vi "补偿电阻RsRp计算.vi"(6 "I":dbl=1.5244, 8 "A":dbl, 9 "压力点个数":dbl=3.0, 10 "检定次数":dbl=1.0, 11 "实时测量数据":string[][](array[string])=[["时间", "温度（℃）", "压力（KPa）", "电压1（V）", "桥压1（V）", "电压2（V）", "桥压2（V）", "电压3（V）", "桥压3（V）", "电压4（V）", "桥压4（V）", "电压5（V）", "桥压5（V）"], ["", "", "1", " ", "2", " ", "3", " ", "4", " ", "", "", ""], ["", "", "正行程", "", "", "", "", "", "", "", "", "", ""], ["17:06:40", "11.900000", "199.921", "-6.32\n-6.32\n", "7.8325\n", "-3.0-6.299\n67000E-6", "-2.844000E-6", "-3.300000E-6", "-3.109000E-6", "-3.045000E-6", "-2.897000E-6", "", ""], ["17:07:13", "12.000000", "299.9351", "51.474", "7.8338", "-3.013000E-6", "-3.491000E-6", "-2.918000E-6", "-3.332000E-6", "-2.780000E-6", "-3.204000E-6", "", ""], ["17:07:36", "12.000000", "399.96", "110.353", "7.8346", "-3.120000E-6", "-3.289000E-6", "-2.960000E-6", "-3.141000E-6", "-3.385000E-6", "-2.844000E-6", "", ""], ["", "", "反行程", "", "", "", "", "", "", "", "", "", ""], ["17:08:20", "12.000000", "400.0285", "110.353", "7.8346", "-3.120000E-6", "-3.342000E-6", "-3.162000E-6", "-3.194000E-6", "-3.056000E-6", "-3.194000E-6", "", ""], ["17:08:45", "12.000000", "300.0653", "52.283", "7.8332", "-3.342000E-6", "-3.321000E-6", "-3.013000E-6", "-3.311000E-6", "-3.300000E-6", "-3.162000E-6", "", ""], ["17:09:22", "12.000000", "200.0595", "-6.299", "7.8346", "-2.907000E-6", "-3.194000E-6", "-3.257000E-6", "-3.204000E-6", "-3.077000E-6", "-2.971000E-6", "", ""], ["", "", "正行程", "", "", "", "", "", "", "", "", "", ""], ["17:13:30", "12.100000", "199.9466", "-7.532", "8.8568", "-3.671000E-6", "-3.353000E-6", "-3.799000E-6", "-3.565000E-6", "-3.746000E-6", "-3.374000E-6", "", ""], ["17:13:53", "12.100000", "299.95", "53.539", "8.8574", "-3.311000E-6", "-3.502000E-6", "-3.364000E-6", "-3.618000E-6", "-3.120000E-6", "-3.406000E-6", "", ""], ["17:14:26", "12.100000", "399.8962", "116.27", "8.8567", "-3.756000E-6", "-3.830000E-6", "-3.427000E-6", "-3.597000E-6", "-3.777000E-6", "-3.576000E-6", "", ""], ["", "", "反行程", "", "", "", "", "", "", "", "", "", ""], ["17:15:01", "12.100000", "399.9835", "116.27", "8.8567", "-3.395000E-6", "-3.289000E-6", "-3.120000E-6", "-3.502000E-6", "-3.427000E-6", "-3.353000E-6", "", ""], ["17:15:38", "12.100000", "299.9459", "54.318", "8.8552", "-3.512000E-6", "-3.650000E-6", "-3.809000E-6", "-3.480000E-6", "-3.300000E-6", "-3.767000E-6", "", ""], ["17:16:15", "12.100000", "199.9841", "-7.516", "8.8564", "-3.629000E-6", "-3.608000E-6", "-3.767000E-6", "-3.639000E-6", "-3.417000E-6", "-3.406000E-6", "", ""]]) -> (1 "Rs":dbl, 2 "Rp":dbl)   [LabVIEW 2017]
uses:
  <vilib>/Analysis/Matrix/Datatypes/RealMatrix.ctl
  676c2c00-1cf9-49e6-a683-8066428fad87.vi
  79778b95-c5f8-4eb7-b08f-402256e2d487.vi
  <vilib>/Array/Sort 2D Array - Pop Stack.vi
  <vilib>/Array/Sort 2D Array - Push Stack.vi
  <vilib>/Analysis/Matrix/NI_Matrix.lvlib
panel:
  out "-40满量程桥压":dbl
  out "-40常压桥压":dbl
  out "-40常压输出":dbl
  out "-40满量程输出":dbl
  out "70满量程桥压":dbl
  out "70常压桥压":dbl
  out "70常压输出":dbl
  out "70满量程输出":dbl
  out "x/y 2":T1 caption="x/y"
  out "x/y":T1
  out "已删除元素的数组子集":string[][](array[string])
  out "70反":dbl[][](array[numeric])
  out "70正":dbl[][](array[numeric])
  out "-40反":dbl[][](array[numeric])
  out "-40正":dbl[][](array[numeric])
  out "70反平均":dbl[][](array[numeric])
  out "70正平均":dbl[][](array[numeric])
  out "-40反平均":dbl[][](array[numeric])
  out "-40正平均":dbl[][](array[numeric])
  in  "数据":dbl[][](array[numeric])=[[199.921, 4.0, 7.8325, 4.0, -2.844e-06, -3.3e-06, -3.109e-06, -3.045e-06, -2.897e-06, 1.0, 0.0], [299.9351, 4.0, 7.8338, 1.0, -3.491e-06, -2.918e-06, -3.332e-06, -2.78e-06, -3.204e-06, 0.0, 0.0], [399.96, 4.0, 7.8346, -3.12e-06, -3.289e-06, -2.96e-06, -3.141e-06, -3.385e-06, -2.844e-06, 0.0, 0.0], [400.0285, -4.0, 7.8346, 0.0, -3.342e-06, -3.162e-06, -3.194e-06, -3.056e-06, -3.194e-06, 0.0, 0.0], [300.0653, -4.0, 7.8332, -3.342e-06, -3.321e-06, -3.013e-06, -3.311e-06, -3.3e-06, -3.162e-06, 0.0, 0.0], [200.0595, -4.0, 7.8346, -2.907e-06, -3.194e-06, -3.257e-06, -3.204e-06, -3.077e-06, -2.971e-06, 0.0, 0.0], [199.9466, 4.0, 8.8568, 5.0, -3.353e-06, -3.799e-06, -3.565e-06, -3.746e-06, -3.374e-06, 0.0, 0.0], [299.95, 4.0, 8.8574, -3.311e-06, -3.502e-06, -3.364e-06, -3.618e-06, -3.12e-06, -3.406e-06, 0.0, 0.0], [399.8962, 4.0, 8.8567, -3.756e-06, -3.83e-06, -3.427e-06, -3.597e-06, -3.777e-06, -3.576e-06, 0.0, 0.0], [399.9835, -4.0, 8.8567, 0.0, -3.289e-06, -3.12e-06, -3.502e-06, -3.427e-06, -3.353e-06, 0.0, 0.0], [299.9459, -4.0, 8.8552, -3.512e-06, -3.65e-06, -3.809e-06, -3.48e-06, -3.3e-06, -3.767e-06, 0.0, 0.0], [199.9841, -4.0, 8.8564, -3.629e-06, -3.608e-06, -3.767e-06, -3.639e-06, -3.417e-06, -3.406e-06, 0.0, 0.0], [200.0, 4.0, 0.0, 1.0, 0.0, 0.0, 0.0, 0.0, 0.0, 0.0, 0.0], [300.0, 4.0, 0.0, 2.0, 0.0, 0.0, 0.0, 0.0, 0.0, 0.0, 0.0], [400.0, 4.0, 0.0, 3.0, 0.0, 0.0, 0.0, 0.0, 0.0, 0.0, 0.0], [400.0, -4.0, 0.0, 20.0, 0.0, 0.0, 0.0, 0.0, 0.0, 0.0, 0.0], [300.0, -4.0, 0.0, 5.0, 0.0, 0.0, 0.0, 0.0, 0.0, 0.0, 0.0], [200.0, -4.0, 0.0, 6.0, 0.0, 0.0, 0.0, 0.0, 0.0, 0.0, 0.0], [200.0, 0.0, 0.0, 7.0, 0.0, 0.0, 0.0, 0.0, 0.0, 0.0, 0.0], [300.0, 0.0, 0.0, 8.0, 0.0, 0.0, 0.0, 0.0, 0.0, 0.0, 0.0], [400.0, 0.0, 0.0, 9.0, 0.0, 0.0, 0.0, 0.0, 0.0, 0.0, 0.0], [400.0, -7.0, 0.0, 10.0, 0.0, 0.0, 0.0, 0.0, 0.0, 0.0, 0.0], [300.0, -7.0, 0.0, 11.0, 0.0, 0.0, 0.0, 0.0, 0.0, 0.0, 0.0], [200.0, -7.0, 0.0, 12.0, 0.0, 0.0, 0.0, 0.0, 0.0, 0.0, 0.0], [0.0, 0.0, 0.0, 13.0, 0.0, 0.0, 0.0, 0.0, 0.0, 0.0, 0.0], [0.0, 0.0, 0.0, 14.0, 0.0, 0.0, 0.0, 0.0, 0.0, 0.0, 0.0], [0.0, 0.0, 0.0, 15.0, 0.0, 0.0, 0.0, 0.0, 0.0, 0.0, 0.0], [0.0, -7.0, 0.0, 16.0, 0.0, 0.0, 0.0, 0.0, 0.0, 0.0, 0.0], [0.0, -7.0, 0.0, 17.0, 0.0, 0.0, 0.0, 0.0, 0.0, 0.0, 0.0], [0.0, -7.0, 0.0, 18.0, 0.0, 0.0, 0.0, 0.0, 0.0, 0.0, 0.0], [0.0, 0.0, 0.0, 19.0, 0.0, 0.0, 0.0, 0.0, 0.0, 0.0, 0.0], [0.0, 0.0, 0.0, 20.0, 0.0, 0.0, 0.0, 0.0, 0.0, 0.0, 0.0], [0.0, 0.0, 0.0, 21.0, 0.0, 0.0, 0.0, 0.0, 0.0, 0.0, 0.0], [0.0, -7.0, 0.0, 22.0, 0.0, 0.0, 0.0, 0.0, 0.0, 0.0, 0.0], [0.0, -7.0, 0.0, 23.0, 0.0, 0.0, 0.0, 0.0, 0.0, 0.0, 0.0], [0.0, -7.0, 0.0, 24.0, 0.0, 0.0, 0.0, 0.0, 0.0, 0.0, 0.0], [0.0, 0.0, 0.0, 25.0, 0.0, 0.0, 0.0, 0.0, 0.0, 0.0, 0.0], [0.0, 0.0, 0.0, 26.0, 0.0, 0.0, 0.0, 0.0, 0.0, 0.0, 0.0], [0.0, 0.0, 0.0, 27.0, 0.0, 0.0, 0.0, 0.0, 0.0, 0.0, 0.0]]
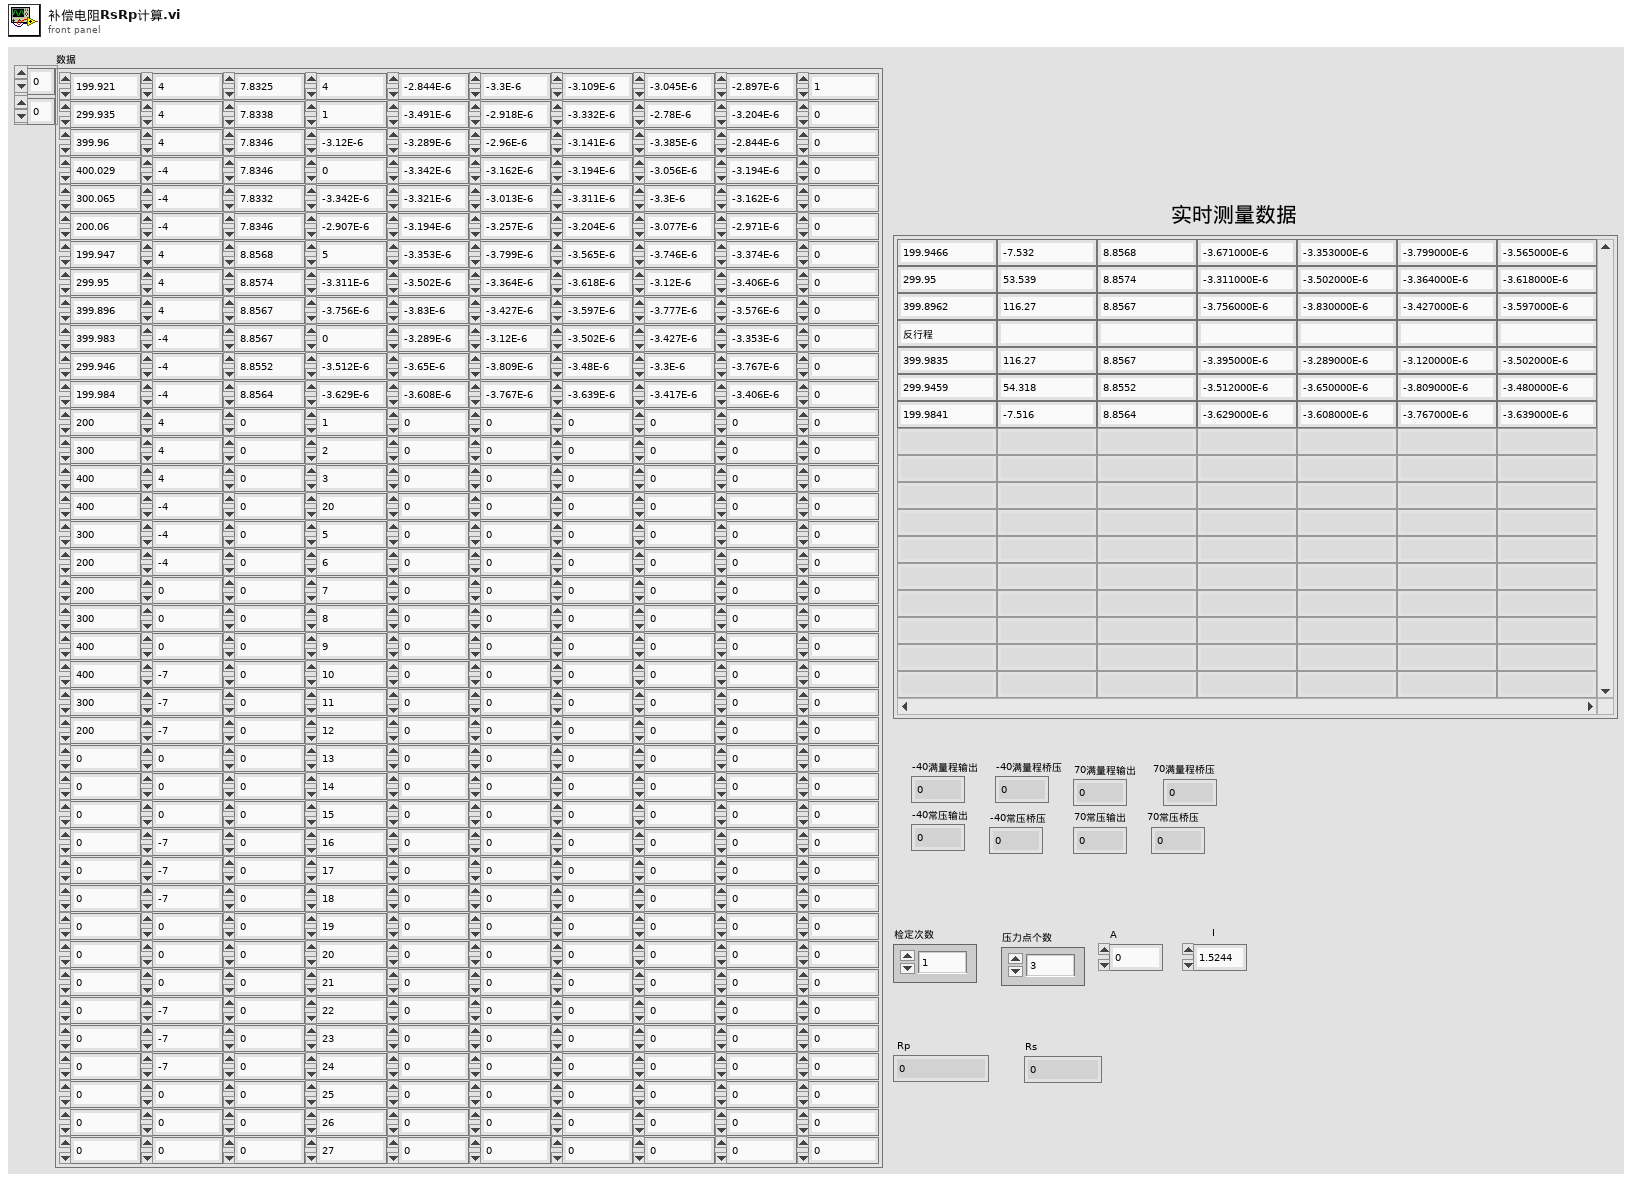
[diagram p1: front panel]
types:
  T1 = typedef "NI_Matrix.lvlib/RealMatrix.ctl" = dbl[][]
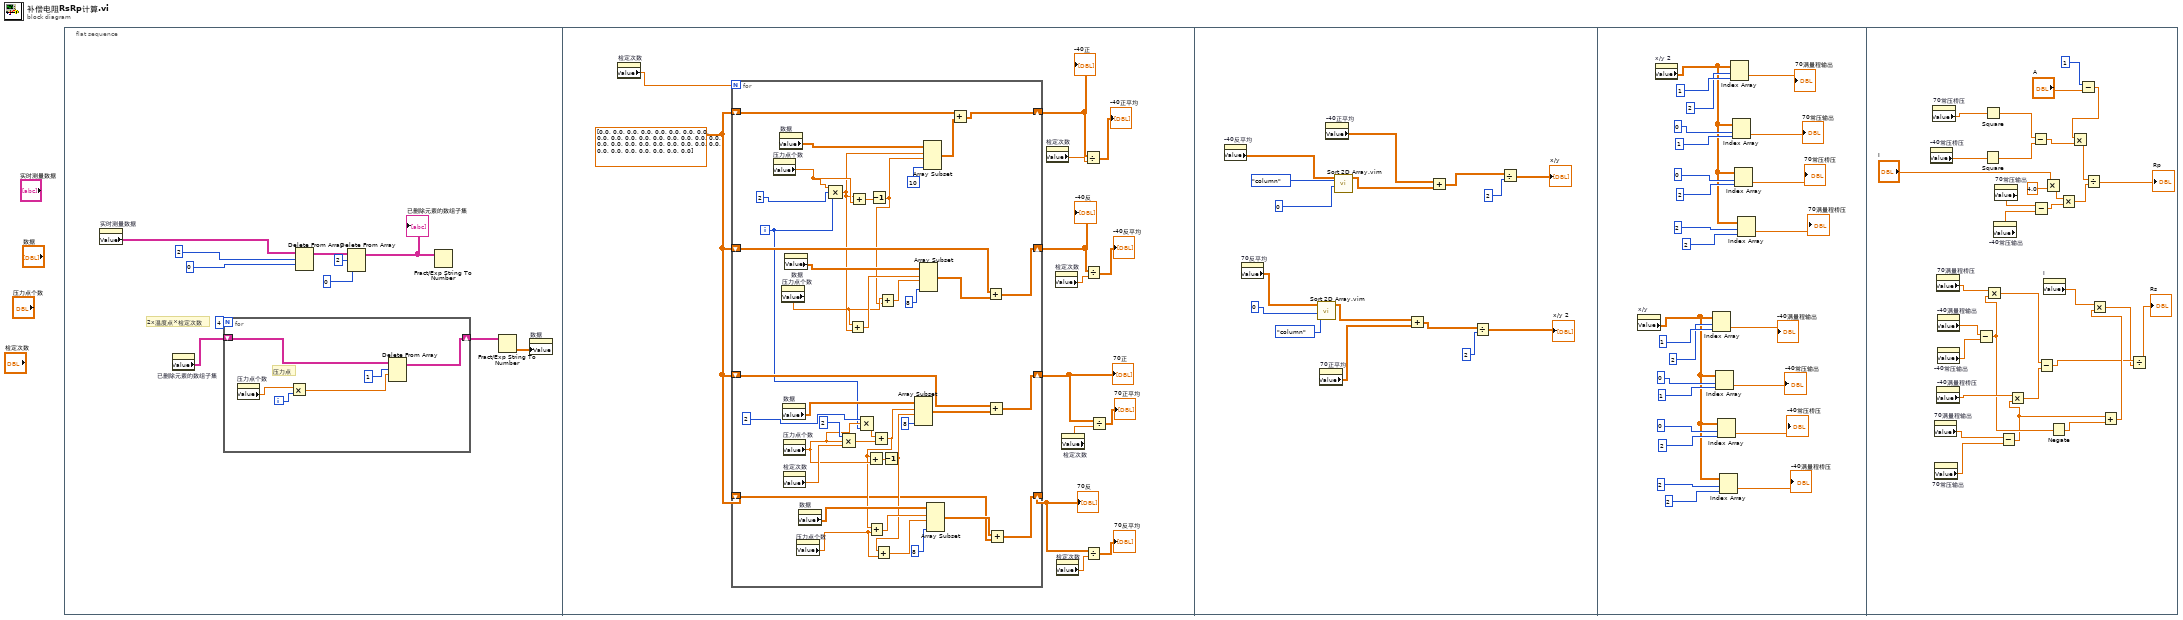
[diagram p0: block diagram]
diagram:
  n1 = flat-sequence {
    frame #0 {
      # "2x温度点×检定次数"
      n2 = property on="实时测量数据" class="Arr (严格)"() -> ("Value"=w9:string[][])  [unwired: 2 in, 2 out]
      n3 = property on="已删除元素的数组子集" class="Arr (严格)"() -> ("Value"=w4:string[][])  [unwired: 2 in, 2 out]
      n4 = for {
        N: 4 -> [_]
        shift-right: [w14] -> w3
        shift-left: w4 -> [w13]
        i -> [w17]
        # "压力点"
        n5 = property on="压力点个数" class="DigNum (严格)"() -> ("Value"=w12:dbl)  [unwired: 2 in, 2 out]
        n6 = Multiply(x=w12, y=w17) -> (x*y=w16:dbl)
        n7 = Delete From Array(array=w13, length=1 ("长度"), index (row)=w16) -> (array with subset deleted=w14:string[][])  [unwired: 1 in, 1 out]
      }
      n8 = Delete From Array(array=w9, length=2 ("长度"), index (row)=0 ("索引 (行)")) -> (array with subset deleted=w8:string[][])  [unwired: 1 in, 1 out]
      n9 = Delete From Array(array=w8, length=2 ("长度"), index (col)=0 ("禁用的索引 (列)")) -> (array with subset deleted=w2:string[][])  [unwired: 1 in, 1 out]
      "已删除元素的数组子集" <- w2
      n10 = Fract/Exp String To Number(string=w2) -> ()  [unwired: 3 in, 2 out]
      n11 = Fract/Exp String To Number(string=w3) -> (number=w1:dbl[][])  [unwired: 3 in, 1 out]
      n12 = property on="数据" class="Arr (严格)"("Value"=w1) -> ()  [unwired: 2 in, 2 out]
    }
    frame #1 {
      w30 = dbl[][] [[0.0, 0.0, 0.0, 0.0, 0.0, 0.0, 0.0, 0.0, 0.0, 0.0, 0.0], [0.0, 0.0, 0.0, 0.0, 0.0, 0.0, 0.0, 0.0, 0.0, 0.0, 0.0], [0.0, 0.0, 0.0, 0.0, 0.0, 0.0, 0.0, 0.0, 0.0, 0.0, 0.0]]
      n13 = property on="检定次数" class="DigNum (严格)"() -> ("Value"=w31:dbl)  [unwired: 2 in, 2 out]
      n14 = for {
        N: w31 -> [_]
        shift-right: [w39] -> w24
        shift-left: w30 -> [w66]
        shift-right: [w38] -> w18
        shift-left: w30 -> [w55]
        shift-right: [w37] -> w19
        shift-left: w30 -> [w46]
        shift-right: [w41] -> w28
        shift-left: w30 -> [w40]
        i -> [w45]
        n15 = property on="压力点个数" class="DigNum (严格)"() -> ("Value"=w44:dbl)  [unwired: 2 in, 2 out]
        n16 = property on="数据" class="Arr (严格)"() -> ("Value"=w72:dbl[][])  [unwired: 2 in, 2 out]
        n17 = property on="压力点个数" class="DigNum (严格)"() -> ("Value"=w33:dbl)  [unwired: 2 in, 2 out]
        n18 = property on="数据" class="Arr (严格)"() -> ("Value"=w65:dbl[][])  [unwired: 2 in, 2 out]
        n19 = property on="压力点个数" class="DigNum (严格)"() -> ("Value"=w57:dbl)  [unwired: 2 in, 2 out]
        n20 = property on="检定次数" class="DigNum (严格)"() -> ("Value"=w62:dbl)  [unwired: 2 in, 2 out]
        n21 = property on="数据" class="Arr (严格)"() -> ("Value"=w68:dbl[][])  [unwired: 2 in, 2 out]
        n22 = property on="压力点个数" class="DigNum (严格)"() -> ("Value"=w50:dbl)  [unwired: 2 in, 2 out]
        n23 = property on="数据" class="Arr (严格)"() -> ("Value"=w54:dbl[][])  [unwired: 2 in, 2 out]
        n24 = Compound Arithmetic op=MULTIPLY(w44, 2, w45) -> (w35:dbl)
        n25 = Compound Arithmetic op=MULTIPLY(2, w57, w62) -> (w58:dbl)
        n26 = Add(x=w33, y=w35) -> (x+y=w36:dbl)
        n27 = Add(x=w35, y=w44) -> (x+y=w70:dbl)
        n28 = Compound Arithmetic op=MULTIPLY(2, w57, w45) -> (w59:dbl)
        n29 = Decrement(x=w70) -> (x-1=w32:dbl)
        n30 = Add(x=w59, y=w58) -> (x+y=w51:dbl)
        n31 = Add(x=w51, y=w57) -> (x+y=w61:dbl)
        n32 = Add(x=w51, y=w50) -> (x+y=w52:dbl)
        n33 = Add(x=w33, y=w32) -> (x+y=w34:dbl)
        n34 = Decrement(x=w61) -> (x-1=w49:dbl)
        n35 = Add(x=w49, y=w50) -> (x+y=w48:dbl)
        n36 = Array Subset(array=w65, index (row)=w51, length (row)=w49, length (col)=8 ("列N")) -> (w56:dbl[][])  [unwired: 1 in]
        n37 = Array Subset(array=w68, index (row)=w36, length (row)=w34, length (col)=8 ("列N")) -> (w67:dbl[][])  [unwired: 1 in]
        n38 = Array Subset(array=w72, index (row)=w35, length (row)=w32, length (col)=10 ("索引 (列)")) -> (w42:dbl[][])  [unwired: 1 in]
        n39 = Array Subset(array=w54, index (row)=w52, length (row)=w48, length (col)=8 ("列N")) -> (w47:dbl[][])  [unwired: 1 in]
        n40 = Add(x=w40, y=w42) -> (x+y=w41:dbl[][])
        n41 = Add(x=w66, y=w67) -> (x+y=w39:dbl[][])
        n42 = Add(x=w55, y=w56) -> (x+y=w38:dbl[][])
        n43 = Add(x=w47, y=w46) -> (x+y=w37:dbl[][])
      }
      "-40正" <- w28
      "-40反" <- w24
      "70正" <- w18
      "70反" <- w19
      n44 = property on="检定次数" class="DigNum (严格)"() -> ("Value"=w29:dbl)  [unwired: 2 in, 2 out]
      n45 = property on="检定次数" class="DigNum (严格)"() -> ("Value"=w26:dbl)  [unwired: 2 in, 2 out]
      n46 = property on="检定次数" class="DigNum (严格)"() -> ("Value"=w21:dbl)  [unwired: 2 in, 2 out]
      n47 = property on="检定次数" class="DigNum (严格)"() -> ("Value"=w22:dbl)  [unwired: 2 in, 2 out]
      n48 = Divide(x=w28, y=w29) -> (x/y=→"-40正平均":dbl[][])
      n49 = Divide(x=w24, y=w26) -> (x/y=→"-40反平均":dbl[][])
      n50 = Divide(x=w19, y=w21) -> (x/y=→"70反平均":dbl[][])
      n51 = Divide(x=w18, y=w22) -> (x/y=→"70正平均":dbl[][])
    }
    frame #2 {
      n52 = property on="-40反平均" class="Arr (严格)"() -> ("Value"=w75:dbl[][])  [unwired: 2 in, 2 out]
      n53 = property on="70反平均" class="Arr (严格)"() -> ("Value"=w73:dbl[][])  [unwired: 2 in, 2 out]
      n54 = call "Sort 2D Array.vim"("index"=0, "dimension to index (column)"=enum16{"column", "row"}."column", "2D array"=w73) -> ("sorted 2D array"=w77:dbl[][])  [unwired: 7 in, 1 out]
      n55 = property on="70正平均" class="Arr (严格)"() -> ("Value"=w74:dbl[][])  [unwired: 2 in, 2 out]
      n56 = property on="-40正平均" class="Arr (严格)"() -> ("Value"=w76:dbl[][])  [unwired: 2 in, 2 out]
      n57 = call "Sort 2D Array.vim"("index"=0, "dimension to index (column)"=enum16{"column", "row"}."column", "2D array"=w75) -> ("sorted 2D array"=w78:dbl[][])  [unwired: 7 in, 1 out]
      n58 = Add ("Add.vi")(x=w77, y=w74) -> (x+y=w84:dbl[][])
      n59 = Add ("Add.vi")(x=w76, y=w78) -> (x+y=w88:dbl[][])
      n60 = Divide(x=w84, y=2) -> (x/y=→"x/y 2":dbl[][])
      n61 = Divide(x=w88, y=2) -> (x/y=→"x/y":dbl[][])
    }
    frame #3 {
      n62 = property on="x/y" class="Arr (严格)"() -> ("Value"=w92:T1)  [unwired: 2 in, 2 out]
      n63 = property on="x/y 2" class="Arr (严格)"() -> ("Value"=w105:T1)  [unwired: 2 in, 2 out]
      n64 = Index Array(array=w92, index (row)=2 ("索引 (行)"), index (col)=1 ("索引 (列)")) -> (element=→"-40满量程输出":dbl)
      n65 = Index Array(array=w92, index (row)=0, index (col)=1 ("索引 (列)")) -> (element=→"-40常压输出":dbl)
      n66 = Index Array(array=w92, index (row)=0 ("索引 (行)"), index (col)=2 ("索引 (列)")) -> (element=→"-40常压桥压":dbl)
      n67 = Index Array(array=w92, index (row)=2 ("索引 (行)"), index (col)=2 ("索引 (列)")) -> (element=→"-40满量程桥压":dbl)
      n68 = Index Array(array=w105, index (row)=2 ("索引 (行)"), index (col)=1 ("索引 (列)")) -> (element=→"70满量程输出":dbl)
      n69 = Index Array(array=w105, index (row)=0, index (col)=1 ("索引 (列)")) -> (element=→"70常压输出":dbl)
      n70 = Index Array(array=w105, index (row)=0 ("索引 (行)"), index (col)=2 ("索引 (列)")) -> (element=→"70常压桥压":dbl)
      n71 = Index Array(array=w105, index (row)=2 ("索引 (行)"), index (col)=2 ("索引 (列)")) -> (element=→"70满量程桥压":dbl)
    }
    frame #4 {
      n72 = property on="-40常压桥压" class="DigNum (严格)"() -> ("Value"=w146:dbl)  [unwired: 2 in, 2 out]
      n73 = property on="70常压桥压" class="DigNum (严格)"() -> ("Value"=w147:dbl)  [unwired: 2 in, 2 out]
      n74 = property on="70满量程输出" class="DigNum (严格)"() -> ("Value"=w116:dbl)  [unwired: 2 in, 2 out]
      n75 = property on="70常压输出" class="DigNum (严格)"() -> ("Value"=w123:dbl)  [unwired: 2 in, 2 out]
      n76 = property on="70满量程桥压" class="DigNum (严格)"() -> ("Value"=w130:dbl)  [unwired: 2 in, 2 out]
      n77 = property on="-40满量程桥压" class="DigNum (严格)"() -> ("Value"=w128:dbl)  [unwired: 2 in, 2 out]
      n78 = property on="-40满量程输出" class="DigNum (严格)"() -> ("Value"=w129:dbl)  [unwired: 2 in, 2 out]
      n79 = property on="-40常压输出" class="DigNum (严格)"() -> ("Value"=w122:dbl)  [unwired: 2 in, 2 out]
      n80 = Subtract(x=w129, y=w122) -> (x-y=w124:dbl)
      n81 = Square(x=w146) -> (x^2=w144:dbl)
      n82 = Square(x=w147) -> (x^2=w145:dbl)
      n83 = Multiply(x=w130, y=w124) -> (x*y=w127:dbl)
      n84 = property on="-40常压输出" class="DigNum (严格)"() -> ("Value"=w141:dbl)  [unwired: 2 in, 2 out]
      n85 = property on="70常压输出" class="DigNum (严格)"() -> ("Value"=w140:dbl)  [unwired: 2 in, 2 out]
      n86 = Subtract(x=w116, y=w123) -> (x-y=w115:dbl)
      n87 = Multiply(x=w128, y=w115) -> (x*y=w126:dbl)
      n88 = Subtract(x=w145, y=w144) -> (x-y=w143:dbl)
      n89 = Subtract(x=w140, y=w141) -> (x-y=w142:dbl)
      n90 = Subtract(x=w127, y=w126) -> (x-y=w119:dbl)
      n91 = property on="I" class="DigNum (严格)"() -> ("Value"=w125:dbl)  [unwired: 2 in, 2 out]
      n92 = Multiply(x="I", y=4.0) -> (x*y=w136:dbl)
      n93 = Negate(x=w124) -> (-x=w121:dbl)
      n94 = Multiply(x=w136, y=w142) -> (x*y=w139:dbl)
      n95 = Subtract(x=1, y="A") -> (x-y=w133:dbl)
      n96 = Multiply(x=w133, y=w143) -> (x*y=w138:dbl)
      n97 = Divide(x=w138, y=w139) -> (x/y=→"Rp":dbl)
      n98 = Add(x=w115, y=w121) -> (x+y=w120:dbl)
      n99 = Multiply(x=w125, y=w120) -> (x*y=w118:dbl)
      n100 = Divide(x=w119, y=w118) -> (x/y=→"Rs":dbl)
    }
  }
